vi "Untitled 3.vi"() -> ()   [LabVIEW 2017]
panel:
  out "X 5":bool=TRUE
  out "X 1":bool=TRUE
  out "X 2":bool=TRUE
  out "X 3":bool=TRUE
  out "X 4":bool=TRUE
  in  "stop 5":bool
  out "Boolean":bool=TRUE
  out "X1":bool=TRUE
  out "X2":bool=TRUE
  out "X3":bool=TRUE
  out "X4":bool=TRUE
  out "X 4":u32=200
  in  "stop 4":bool
  out "X=2":bool=TRUE
  out "X=4":bool=TRUE
  out "X=6":bool=TRUE
  out "X=8":bool=TRUE
  out "X 3":u32=200
  in  "stop 3":bool
  out "X= 2":bool=TRUE
  out "X=4":bool=TRUE
  out "X=6":bool=TRUE
  out "X=8":bool=TRUE
  out "X 2":u32=200
  in  "stop 2":bool
  in  "stop":bool
  out "X":u32=200
  out "X=8":bool=TRUE
  out "X=6":bool=TRUE
  out "X=4":bool=TRUE
  out "X=2":bool=TRUE
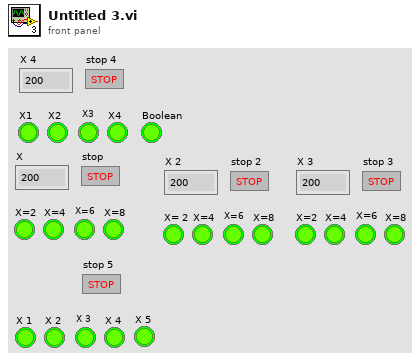
[diagram p1: front panel]
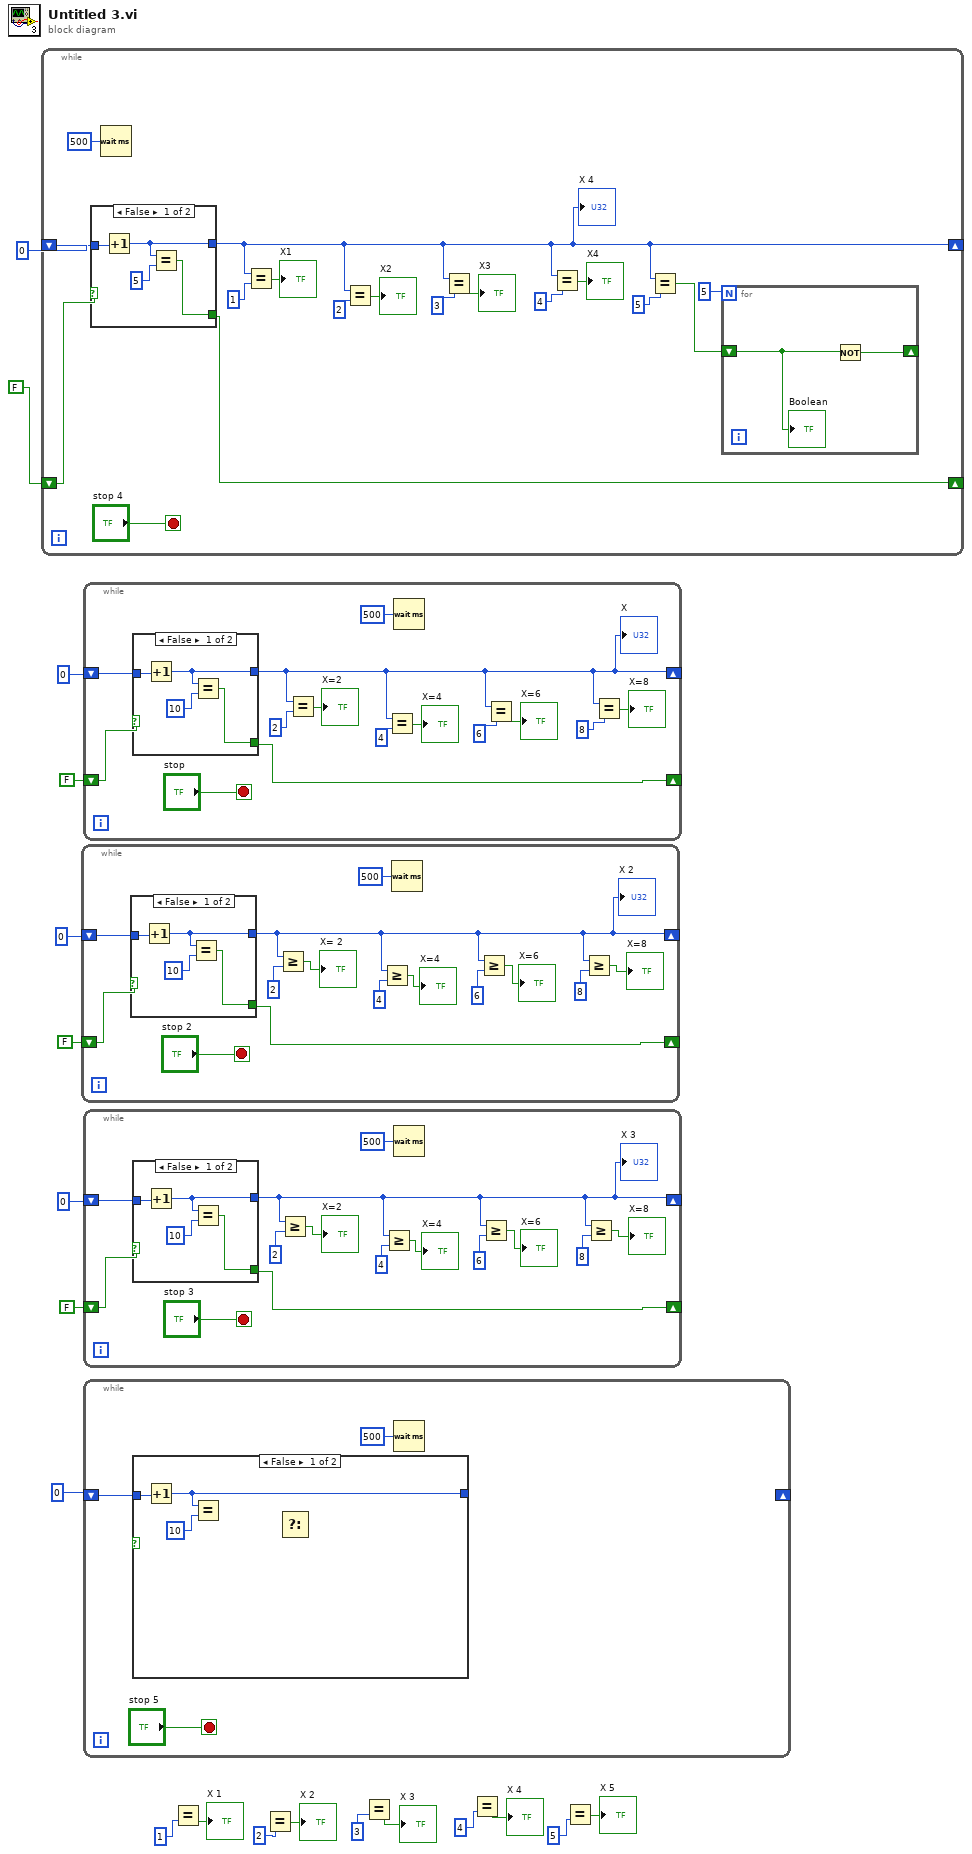
[diagram p0: block diagram]
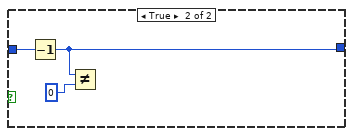
[diagram p2: hidden frame]
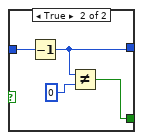
[diagram p3: hidden frame]
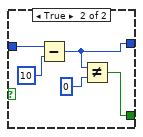
[diagram p4: hidden frame]
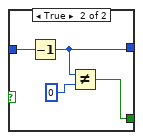
[diagram p5: hidden frame]
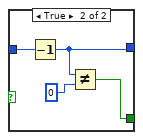
[diagram p6: hidden frame]
diagram:
  n1 = while {
    shift-right: [w22] -> _
    shift-left: u32 0 ("milliseconds to wait") -> [w35]
    shift-right: [w33] -> _
    shift-left: FALSE -> [w34]
    stop <- "stop 4" stop-if-true
    n2 = case shown="False" w34 {
      tunnel: w35 -> [w42 w46]
      tunnel: [w40 w45] -> w22
      tunnel: [w39 w43] -> w33
      frame False {
        n3 = Increment(x=w42) -> (x+1=w40:u32)
        n4 = Equal?(x=w40, y=u32 5 ("milliseconds to wait")) -> (x = y?=w39:bool)
      }
      frame True {
        n5 = Decrement(x=w46) -> (x-1=w45:u32)
        n6 = Not Equal?(x=w45, y=u32 0 ("milliseconds to wait")) -> (x != y?=w43:bool)
      }
    }
    "X 4" <- w22
    n7 = Wait (ms)(milliseconds to wait=u32 500) -> ()  [unwired: 1 out]
    n8 = Equal?(x=w22, y=u32 1 ("milliseconds to wait")) -> (x = y?=→"X1":bool)
    n9 = Equal?(x=w22, y=u32 2 ("milliseconds to wait")) -> (x = y?=→"X2":bool)
    n10 = Equal?(x=w22, y=u32 3 ("milliseconds to wait")) -> (x = y?=→"X3":bool)
    n11 = Equal?(x=w22, y=u32 4 ("milliseconds to wait")) -> (x = y?=→"X4":bool)
    n12 = Equal?(x=w22, y=u32 5 ("milliseconds to wait")) -> (x = y?=w20:bool)
    n13 = for {
      N: u32 5 ("milliseconds to wait") -> [_]
      shift-right: [w38] -> _
      shift-left: w20 -> [w37]
      n14 = Not(x=w37) -> (.not. x?=w38:bool)
      "Boolean" <- w37
    }
  }
  n15 = while {
    shift-right: [w49] -> _
    shift-left: u32 0 ("milliseconds to wait") -> [w59]
    shift-right: [w57] -> _
    shift-left: FALSE -> [w58]
    stop <- "stop 2" stop-if-true
    n16 = case shown="False" w58 {
      tunnel: w59 -> [w64 w68]
      tunnel: [w62 w67] -> w49
      tunnel: [w61 w65] -> w57
      frame False {
        n17 = Increment(x=w64) -> (x+1=w62:u32)
        n18 = Equal?(x=w62, y=u32 10 ("milliseconds to wait")) -> (x = y?=w61:bool)
      }
      frame True {
        n19 = Decrement(x=w68) -> (x-1=w67:u32)
        n20 = Not Equal?(x=w67, y=u32 0 ("milliseconds to wait")) -> (x != y?=w65:bool)
      }
    }
    "X 2" <- w49
    n21 = Greater Or Equal?(x=w49, y=u32 2 ("milliseconds to wait")) -> (x >= y?=→"X= 2":bool)
    n22 = Greater Or Equal?(x=w49, y=u32 4 ("milliseconds to wait")) -> (x >= y?=→"X=4":bool)
    n23 = Wait (ms)(milliseconds to wait=u32 500) -> ()  [unwired: 1 out]
    n24 = Greater Or Equal?(x=w49, y=u32 6 ("milliseconds to wait")) -> (x >= y?=→"X=6":bool)
    n25 = Greater Or Equal?(x=w49, y=u32 8 ("milliseconds to wait")) -> (x >= y?=→"X=8":bool)
  }
  n26 = while {
    shift-right: [w70] -> _
    shift-left: u32 0 ("milliseconds to wait") -> [w81]
    shift-right: [w79] -> _
    shift-left: FALSE -> [w80]
    stop <- "stop" stop-if-true
    n27 = case shown="False" w80 {
      tunnel: w81 -> [w86 w90]
      tunnel: [w84 w89] -> w70
      tunnel: [w83 w87] -> w79
      frame False {
        n28 = Increment(x=w86) -> (x+1=w84:u32)
        n29 = Equal?(x=w84, y=u32 10 ("milliseconds to wait")) -> (x = y?=w83:bool)
      }
      frame True {
        n30 = Decrement(x=w90) -> (x-1=w89:u32)
        n31 = Not Equal?(x=w89, y=u32 0 ("milliseconds to wait")) -> (x != y?=w87:bool)
      }
    }
    "X" <- w70
    n32 = Equal?(x=w70, y=u32 2 ("milliseconds to wait")) -> (x = y?=→"X=2":bool)
    n33 = Equal?(x=w70, y=u32 4 ("milliseconds to wait")) -> (x = y?=→"X=4":bool)
    n34 = Wait (ms)(milliseconds to wait=u32 500) -> ()  [unwired: 1 out]
    n35 = Equal?(x=w70, y=u32 6 ("milliseconds to wait")) -> (x = y?=→"X=6":bool)
    n36 = Equal?(x=w70, y=u32 8 ("milliseconds to wait")) -> (x = y?=→"X=8":bool)
  }
  n37 = while {
    shift-right: [w93] -> _
    shift-left: u32 0 ("milliseconds to wait") -> [w103]
    shift-right: [w101] -> _
    shift-left: FALSE -> [w102]
    stop <- "stop 3" stop-if-true
    n38 = case shown="False" w102 {
      tunnel: w103 -> [w108 w113]
      tunnel: [w106 w110] -> w93
      tunnel: [w105 w109] -> w101
      frame False {
        n39 = Increment(x=w108) -> (x+1=w106:u32)
        n40 = Equal?(x=w106, y=u32 10 ("milliseconds to wait")) -> (x = y?=w105:bool)
      }
      frame True {
        n41 = Subtract(x=w113, y=u32 10 ("milliseconds to wait")) -> (x-y=w110:u32)
        n42 = Not Equal?(x=w110, y=u32 0 ("milliseconds to wait")) -> (x != y?=w109:bool)
      }
    }
    "X 3" <- w93
    n43 = Greater Or Equal?(x=w93, y=u32 2 ("milliseconds to wait")) -> (x >= y?=→"X=2":bool)
    n44 = Greater Or Equal?(x=w93, y=u32 4 ("milliseconds to wait")) -> (x >= y?=→"X=4":bool)
    n45 = Wait (ms)(milliseconds to wait=u32 500) -> ()  [unwired: 1 out]
    n46 = Greater Or Equal?(x=w93, y=u32 6 ("milliseconds to wait")) -> (x >= y?=→"X=6":bool)
    n47 = Greater Or Equal?(x=w93, y=u32 8 ("milliseconds to wait")) -> (x >= y?=→"X=8":bool)
  }
  n48 = while {
    shift-right: _ -> [_]
    shift-left: u32 0 ("milliseconds to wait") -> [w115]
    stop <- "stop 5" stop-if-true
    n49 = case shown="False" {
      selector: _ -> [_ _]
      tunnel: w115 -> [w119 w123]
      tunnel: [w117 w122] -> _
      frame False {
        n50 = Increment(x=w119) -> (x+1=w117:u32)
        n51 = Equal?(x=w117, y=u32 10 ("milliseconds to wait")) -> ()  [unwired: 1 out]
        n52 = Select() -> ()  [unwired: 3 in, 1 out]
      }
      frame True {
        n53 = Decrement(x=w123) -> (x-1=w122:u32)
        n54 = Not Equal?(x=w122, y=u32 0 ("milliseconds to wait")) -> (x != y?=w120:bool)
      }
    }
    n55 = Wait (ms)(milliseconds to wait=u32 500) -> ()  [unwired: 1 out]
  }
  n56 = Equal?(y=u32 1 ("milliseconds to wait")) -> (x = y?=→"X 1":bool)  [unwired: 1 in]
  n57 = Equal?(y=u32 2 ("milliseconds to wait")) -> (x = y?=→"X 2":bool)  [unwired: 1 in]
  n58 = Equal?(y=u32 3 ("milliseconds to wait")) -> (x = y?=→"X 3":bool)  [unwired: 1 in]
  n59 = Equal?(y=u32 4 ("milliseconds to wait")) -> (x = y?=→"X 4":bool)  [unwired: 1 in]
  n60 = Equal?(y=u32 5 ("milliseconds to wait")) -> (x = y?=→"X 5":bool)  [unwired: 1 in]
